vi "Write Voltage Data to Optimization.vi"(5 "Network Data Array":T1[](array[typedef]), 7 "Bus by ID":T2[](array[typedef]), 8 "error in":errorcluster, 11 "Generic Optimization in":refnum<class "Generic Optimization.lvclass">) -> (0 "error out":errorcluster, 3 "Generic Optimization out":refnum<class "Generic Optimization.lvclass">)   [LabVIEW 2018, in "Generic Optimization Actor.lvlib" / "Generic Optimization.lvclass"]
uses:
  Generic Optimization.lvclass
  C:/Users/Administrator/Desktop/LabVIEW EMS/EMS Generic Actor/EMS Generic/EMS Generic.lvclass
  Optimization Controls/Bus by ID.ctl
  <vilib>/ORNL/CSEISMIC DDS/CSEISMIC DDS Base/Data Types/Controls/DeviceID.ctl
  Optimization Controls/Electrical Network Optimization Data.ctl
  EMS Generic Actor/EMS Generic/EMS Generic.lvclass/EMS Generic.ctl
  Optimization Controls/Bus Voltage.ctl
  <vilib>/ORNL/CSEISMIC DDS/CSEISMIC DDS Base/Data Types/SmartRelay_Measurement.ctl
  <vilib>/ORNL/CSEISMIC DDS/CSEISMIC DDS Base/Data Types/DER_Measurement.ctl
  <vilib>/ORNL/CSEISMIC DDS/CSEISMIC DDS Base/Data Types/Meter_Measurement.ctl
  Global Variables/Global Variables.vi
  <vilib>/ORNL/CSEISMIC DDS/CSEISMIC DDS Base/CSEISMIC DDS.lvclass
  EMS Generic Actor/EMS Generic/EMS Generic.lvclass
  <vilib>/Analysis/NI_AALBase.lvlib
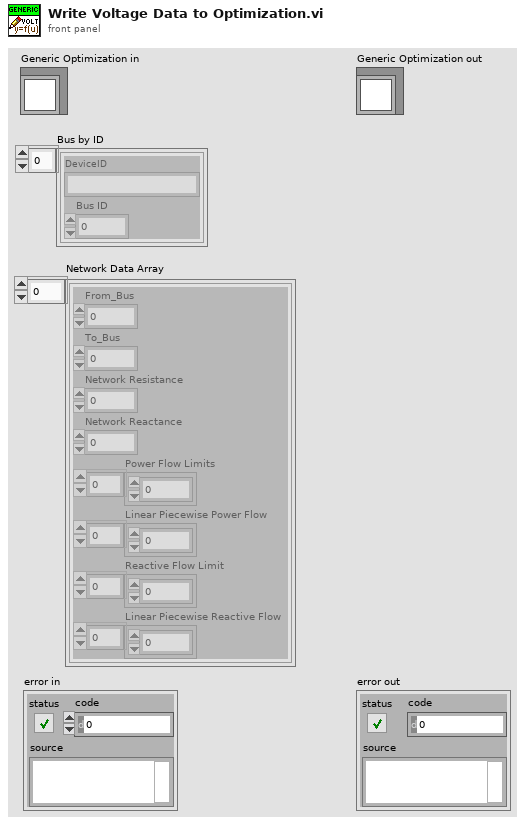
[diagram p1: front panel]
types:
  T1 = typedef "Generic Optimization Actor.lvlib/Generic Optimization.lvclass/Electrical Network Optimization Data.ctl" = cluster{"From_Bus":dbl, "To_Bus":dbl, "Network Resistance":dbl, "Network Reactance":dbl, "Power Flow Limits":dbl[], "Linear Piecewise Power Flow":dbl[], "Reactive Flow Limit":dbl[], "Linear Piecewise Reactive Flow":dbl[]}
  T2 = typedef "Generic Optimization Actor.lvlib/Generic Optimization.lvclass/Bus by ID.ctl" = cluster{"DeviceID":T3, "Bus ID":dbl}
  T3 = typedef "CSEISMIC DDS.lvlib/CSEISMIC DDS.lvclass/DeviceID.ctl" = string
  T4 = typedef "Generic Optimization Actor.lvlib/Generic Optimization.lvclass/Bus Voltage.ctl" = cluster{"Bus":dbl, "Voltage":dbl}
  T5 = typedef "CSEISMIC DDS.lvlib/CSEISMIC DDS.lvclass/Meter_Measurement.ctl" = cluster{"DeviceID":T3, "Voltage":dbl[], "Current":dbl[], "RealPower":dbl[], "ReactivePower":dbl[], "LineConfig":u8[], "Frequency":dbl}
  T6 = typedef "CSEISMIC DDS.lvlib/CSEISMIC DDS.lvclass/SmartRelay_Measurement.ctl" = cluster{"DeviceID":T3, "PrimaryVoltage":dbl[], "SecondaryVoltage":dbl[], "Current":dbl[], "RealPower":dbl[], "ReactivePower":dbl[], "LineConfig":u8[], "Frequency":dbl}
  T7 = typedef "CSEISMIC DDS.lvlib/CSEISMIC DDS.lvclass/DER_Measurement.ctl" = cluster{"DeviceID":T3, "Voltage":dbl[], "Current":dbl[], "RealPower":dbl[], "ReactivePower":dbl[], "LineConfig":u8[], "Frequency":dbl}
  T8 = typedef "EMS Generic Actor.lvlib/EMS Generic.lvclass/Data Type DVRs.ctl" = cluster{"IED_Status":refnum<data-value>, "IED_Status_0":refnum<data-value>, "DER_Measurement":refnum<data-value>, "DER_Info":refnum<data-value>, "DER_Status":refnum<data-value>, "ES_Measurement":refnum<data-value>, "ES_Info":refnum<data-value>, "PV_Info":refnum<data-value>, "SmartRelay_Info":refnum<data-value>, "SmartRelay_Measurement":refnum<data-value>, "Meter_Info":refnum<data-value>, "Meter_Measurement":refnum<data-value>, "HVAC_Status":refnum<data-value>, "HVAC_Measurement":refnum<data-value>, "PriceData_RealTime":refnum<data-value>, "PriceData_Demand":refnum<data-value>, "PriceData_Energy":refnum<data-value>, "ForecastData_Long":refnum<data-value>, "ForecastData_Short":refnum<data-value>, "DER_Control":refnum<data-value>, "DER_SetPointF":refnum<data-value>, "DER_SetPointP":refnum<data-value>, "DER_SetPointQ":refnum<data-value>, "DER_SetPointPF":refnum<data-value>, "DER_SetPointV":refnum<data-value>, "PV_setCurtailment":refnum<data-value>, "PV_setRampRate":refnum<data-value>, "Relay_Control":refnum<data-value>, "Load_Control":refnum<data-value>, "HVAC_Control":refnum<data-value>, "Generator_Info":refnum<data-value>, "ForecastData_Long_Backup":refnum<data-value>, "PriceData_RealTime_Backup":refnum<data-value>}
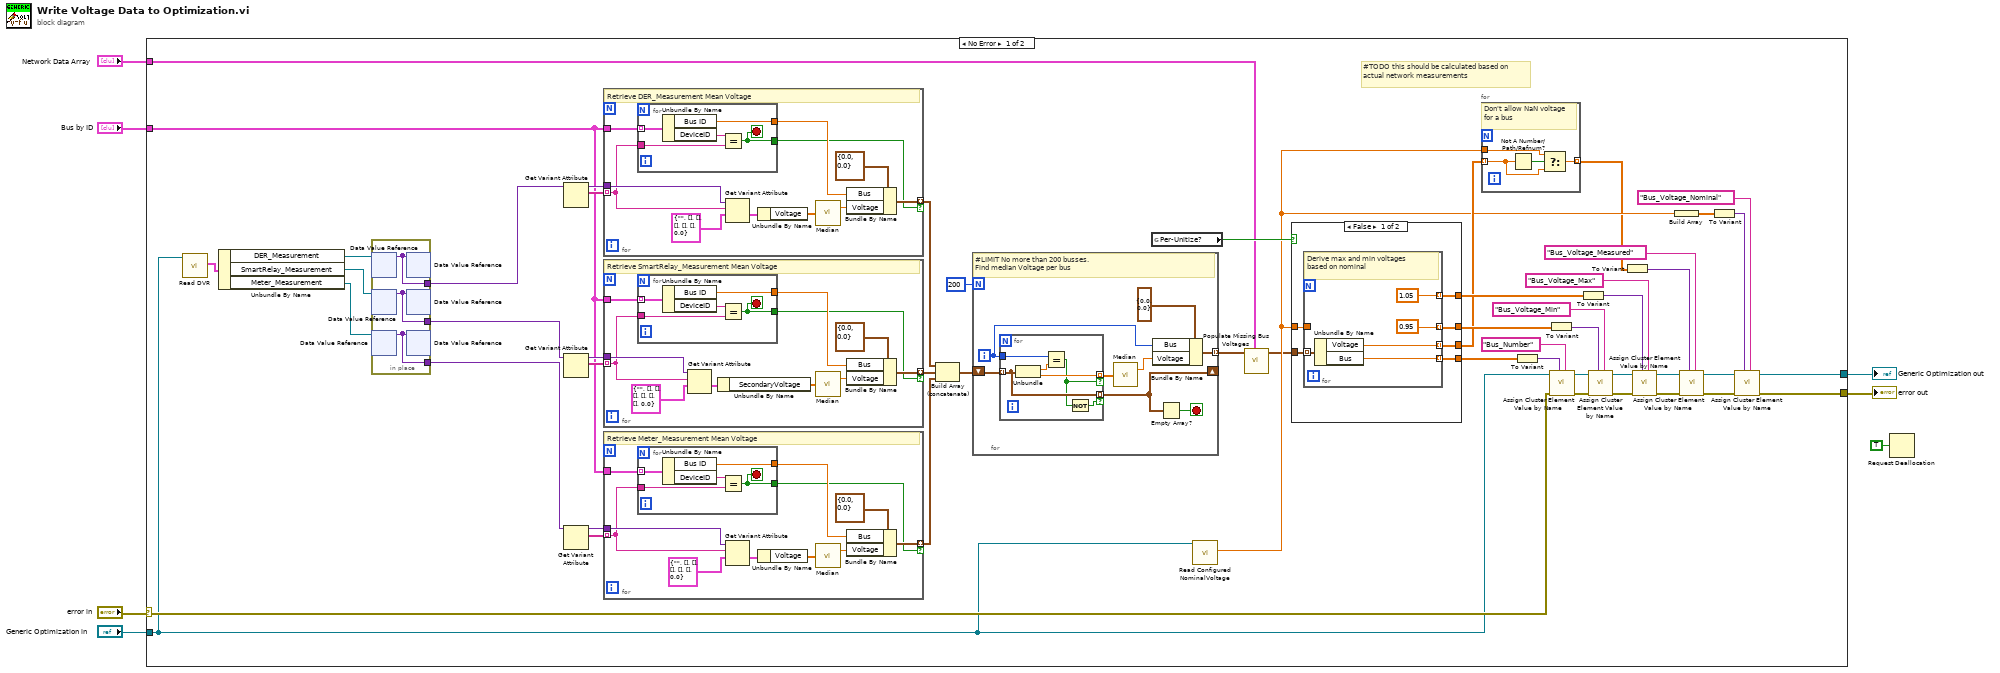
[diagram p0: block diagram]
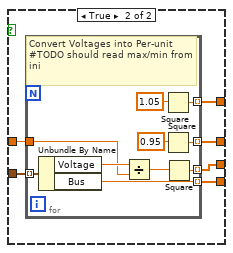
[diagram p2: hidden frame]
diagram:
  n1 = case shown="No Error" "error in" {
    selector: "error in" -> [w45 w157]
    tunnel: [w20 w157] -> w7
    tunnel: "Bus by ID" -> [w27 _]
    tunnel: "Generic Optimization in" -> [w9 w156]
    tunnel: [w8 w156] -> w3
    tunnel: "Network Data Array" -> [w10 _]
    frame No Error {
      # "#TODO this should be calculated based on actual network measurements"
      n2 = call "Read DVR.vi"("EMS Generic in"=w9) -> ("DVR"=w41:T8)  [unwired: 9 in, 1 out]
      n3 = Unbundle By Name(w41) -> ("DER_Measurement"=w40:refnum<data-value>, "SmartRelay_Measurement"=w39:refnum<data-value>, "Meter_Measurement"=w26:refnum<data-value>)
      n4 = in-place {
        in-place-border: [w155] -> w25
        in-place-border: [w154] -> w24
        in-place-border: [w153] -> w23
        n5 = in-place-dvr #1(w40) -> (w155:variant)  [unwired: 1 out]
        n6 = in-place-dvr #2(w39) -> (w154:variant)  [unwired: 1 out]
        n7 = in-place-dvr #3(w26) -> (w153:variant)  [unwired: 1 out]
        n8 = in-place-dvr #1(w155) -> ()  [unwired: 2 out]
        n9 = in-place-dvr #2(w154) -> ()  [unwired: 2 out]
        n10 = in-place-dvr #3(w153) -> ()  [unwired: 2 out]
      }
      n11 = Get Variant Attribute(Variant=w25) -> (duplicate Variant=w37:variant, names=w38:string[])  [unwired: 3 in, 2 out]
      n12 = Get Variant Attribute(Variant=w24) -> (duplicate Variant=w36:variant, names=w35:string[])  [unwired: 3 in, 2 out]
      n13 = Get Variant Attribute(Variant=w23) -> (duplicate Variant=w33:variant, names=w34:string[])  [unwired: 3 in, 2 out]
      n14 = for {
        tunnel: w38 -> [w145] mode=indexing
        tunnel: w37 -> [w147]
        tunnel: w27 -> [w146]
        tunnel: [w143] -> w32 mode=indexing if=w137
        # "Retrieve DER_Measurement Mean Voltage"
        n15 = for {
          tunnel: w146 -> [w152] mode=indexing
          tunnel: w145 -> [w151]
          tunnel: [w149] -> w139
          tunnel: [w148] -> w137
          stop <- w148 stop-if-true
          n16 = Unbundle By Name(w152) -> ("Bus ID"=w149:dbl, "DeviceID"=w150:T3)
          n17 = Equal?(x=w150, y=w151) -> (x = y?=w148:bool)
        }
        n18 = Get Variant Attribute(Variant=w147, name=w145, default value (empty Variant)=T7 {"DeviceID"="", "Voltage"=[], "Current"=[], "RealPower"=[], "ReactivePower"=[], "LineConfig"=[], "Frequency"=0.0} ("DER_Measurement")) -> (value=w144:T7)  [unwired: 1 in, 3 out]
        n19 = Unbundle By Name(w144) -> ("Voltage"=w141:dbl[])
        n20 = call <vilib>:"Median.vi"("X"=w141) -> ("median"=w140:dbl)  [unwired: 1 out]
        n21 = Bundle By Name(cluster=T4 {"Bus"=0.0, "Voltage"=0.0} ("Bus Voltage"), "Bus"=w139, "Voltage"=w140) -> (w143:T4)
      }
      n22 = for {
        tunnel: w35 -> [w129] mode=indexing
        tunnel: w36 -> [w131]
        tunnel: w27 -> [w130]
        tunnel: [w127] -> w31 mode=indexing if=w122
        # "Retrieve SmartRelay_Measurement Mean Voltage"
        n23 = for {
          tunnel: w130 -> [w136] mode=indexing
          tunnel: w129 -> [w135]
          tunnel: [w133] -> w124
          tunnel: [w132] -> w122
          stop <- w132 stop-if-true
          n24 = Unbundle By Name(w136) -> ("Bus ID"=w133:dbl, "DeviceID"=w134:T3)
          n25 = Equal?(x=w134, y=w135) -> (x = y?=w132:bool)
        }
        n26 = Get Variant Attribute(Variant=w131, name=w129, default value (empty Variant)=T6 {"DeviceID"="", "PrimaryVoltage"=[], "SecondaryVoltage"=[], "Current"=[], "RealPower"=[], "ReactivePower"=[], "LineConfig"=[], "Frequency"=0.0} ("SmartRelay_Measurement")) -> (value=w128:T6)  [unwired: 1 in, 3 out]
        n27 = Unbundle By Name(w128) -> ("SecondaryVoltage"=w126:dbl[])
        n28 = call <vilib>:"Median.vi"("X"=w126) -> ("median"=w125:dbl)  [unwired: 1 out]
        n29 = Bundle By Name(cluster=T4 {"Bus"=0.0, "Voltage"=0.0} ("Bus Voltage"), "Bus"=w124, "Voltage"=w125) -> (w127:T4)
      }
      n30 = for {
        tunnel: w34 -> [w113] mode=indexing
        tunnel: w33 -> [w115]
        tunnel: w27 -> [w114]
        tunnel: [w111] -> w30 mode=indexing if=w106
        # "Retrieve Meter_Measurement Mean Voltage"
        n31 = for {
          tunnel: w114 -> [w120] mode=indexing
          tunnel: w113 -> [w119]
          tunnel: [w117] -> w108
          tunnel: [w116] -> w106
          stop <- w116 stop-if-true
          n32 = Unbundle By Name(w120) -> ("Bus ID"=w117:dbl, "DeviceID"=w118:T3)
          n33 = Equal?(x=w118, y=w119) -> (x = y?=w116:bool)
        }
        n34 = Get Variant Attribute(Variant=w115, name=w113, default value (empty Variant)=T5 {"DeviceID"="", "Voltage"=[], "Current"=[], "RealPower"=[], "ReactivePower"=[], "LineConfig"=[], "Frequency"=0.0} ("Meter_Measurement")) -> (value=w112:T5)  [unwired: 1 in, 3 out]
        n35 = Unbundle By Name(w112) -> ("Voltage"=w110:dbl[])
        n36 = call <vilib>:"Median.vi"("X"=w110) -> ("median"=w109:dbl)  [unwired: 1 out]
        n37 = Bundle By Name(cluster=T4 {"Bus"=0.0, "Voltage"=0.0} ("Bus Voltage"), "Bus"=w108, "Voltage"=w109) -> (w111:T4)
      }
      n38 = Build Array (concatenate)(w32, w31, w30) -> (w29:T4[])
      n39 = for {
        N: 200 -> [_]
        shift-right: [w97] -> _
        shift-left: w29 -> [w98]
        tunnel: [w93] -> w12 mode=indexing
        i -> [w94]
        stop <- w96 stop-if-true
        # "#LIMIT No more than 200 busses.\nFind median Voltage per bus"
        n40 = for {
          tunnel: w98 -> [w101] mode=indexing
          tunnel: w94 -> [w104]
          tunnel: [w102] -> w92 mode=indexing if=w100
          tunnel: [w101] -> w97 mode=indexing if=w99
          n41 = Unbundle(w101) -> ("Bus"=w103:dbl, "Voltage"=w102:dbl)
          n42 = Equal?(x=w104, y=w103) -> (x = y?=w100:bool)
          n43 = Not(x=w100) -> (.not. x?=w99:bool)
        }
        n44 = call <vilib>:"Median.vi"("X"=w92) -> ("median"=w91:dbl)  [unwired: 1 out]
        n45 = Bundle By Name(cluster=T4 {"Bus"=0.0, "Voltage"=0.0} ("Bus Voltage"), "Bus"=w94, "Voltage"=w91) -> (w93:T4)
        n46 = Empty Array?(array=w97) -> (empty?=w96:bool)
      }
      n47 = global read "Global Variables.vi" "Per-Unitize?"() -> (w22:bool)
      n48 = call "Read Configured NominalVoltage.vi"("EMS Generic in"=w9) -> ("NominalVoltage"=w14:dbl)  [unwired: 8 in, 2 out]
      n49 = call "Populate Missing Bus Voltages.vi"("Network Data Array"=w10, "Bus Voltage Array in"=w12) -> ("Bus Voltage Array out"=w11:T4[])  [unwired: 8 in, 1 out]
      n50 = case shown="False" w22 {
        tunnel: [w69 w75] -> w44
        tunnel: [w68 w77] -> w43
        tunnel: [w67 w78] -> w42
        tunnel: [w66 w76] -> w15
        tunnel: w11 -> [w65 w79]
        tunnel: w14 -> [w64 w80]
        frame False {
          n51 = for {
            tunnel: w65 -> [w74] mode=indexing
            tunnel: [w72] -> w66 mode=indexing
            tunnel: w64 -> [_]
            tunnel: [1.05] -> w67 mode=indexing
            tunnel: [0.95] -> w68 mode=indexing
            tunnel: [w73] -> w69 mode=indexing
            # "Derive max and min voltages based on nominal"
            n52 = Unbundle By Name(w74) -> ("Voltage"=w72:dbl, "Bus"=w73:dbl)
          }
        }
        frame True {
          n53 = for {
            tunnel: w79 -> [w90] mode=indexing
            tunnel: [w89] -> w76 mode=indexing
            tunnel: w80 -> [w84]
            tunnel: [w88] -> w78 mode=indexing
            tunnel: [w87] -> w77 mode=indexing
            tunnel: [w86] -> w75 mode=indexing
            # "Convert Voltages into Per-unit\n#TODO should read max/min from ini"
            n54 = Unbundle By Name(w90) -> ("Voltage"=w85:dbl, "Bus"=w86:dbl)
            n55 = Divide(x=w85, y=w84) -> (x/y=w81:dbl)
            n56 = Square(x=1.05) -> (x^2=w88:dbl)
            n57 = Square(x=0.95) -> (x^2=w87:dbl)
            n58 = Square(x=w81) -> (x^2=w89:dbl)
          }
        }
      }
      n59 = for {
        tunnel: w15 -> [w62] mode=indexing
        tunnel: w14 -> [w61]
        tunnel: [w60] -> w13 mode=indexing
        # "Don't allow NaN voltage for a bus"
        n60 = Not A Number/Path/Refnum?(number/path/refnum=w62) -> (NaN/Path/Refnum?=w63:bool)
        n61 = Select(t=w61, s=w63, f=w62) -> (s? t:f=w60:dbl)
      }
      n62 = To Variant(anything=w44) -> (Variant=w46:variant)
      n63 = To Variant(anything=w43) -> (Variant=w48:variant)
      n64 = call "Assign Cluster Element Value by Name.vi"("Element Name"="Bus_Number" ("Keyword Name"), "Value"=w46, "error in"=w45, "Generic Optimization"=w9) -> ("error out"=w57:errorcluster, "Generic Optimization out"=w56:refnum<class "Generic Optimization.lvclass">)  [unwired: 6 in]
      n65 = To Variant(anything=w42) -> (Variant=w50:variant)
      n66 = call "Assign Cluster Element Value by Name.vi"("Element Name"="Bus_Voltage_Min" ("Keyword Name"), "Value"=w48, "error in"=w57, "Generic Optimization"=w56) -> ("error out"=w58:errorcluster, "Generic Optimization out"=w55:refnum<class "Generic Optimization.lvclass">)  [unwired: 6 in]
      n67 = To Variant(anything=w13) -> (Variant=w52:variant)
      n68 = call "Assign Cluster Element Value by Name.vi"("Element Name"="Bus_Voltage_Max" ("Keyword Name"), "Value"=w50, "error in"=w58, "Generic Optimization"=w55) -> ("error out"=w59:errorcluster, "Generic Optimization out"=w54:refnum<class "Generic Optimization.lvclass">)  [unwired: 6 in]
      n69 = Build Array(w14) -> (w16:dbl[])
      n70 = call "Assign Cluster Element Value by Name.vi"("Element Name"="Bus_Voltage_Measured" ("Keyword Name"), "Value"=w52, "error in"=w59, "Generic Optimization"=w54) -> ("error out"=w21:errorcluster, "Generic Optimization out"=w19:refnum<class "Generic Optimization.lvclass">)  [unwired: 6 in]
      n71 = To Variant(anything=w16) -> (Variant=w18:variant)
      n72 = call "Assign Cluster Element Value by Name.vi"("Element Name"="Bus_Voltage_Nominal" ("Keyword Name"), "Value"=w18, "error in"=w21, "Generic Optimization"=w19) -> ("error out"=w20:errorcluster, "Generic Optimization out"=w8:refnum<class "Generic Optimization.lvclass">)  [unwired: 6 in]
    }
    frame Error {
    }
  }
  "error out" <- w7
  "Generic Optimization out" <- w3
  n73 = Request Deallocation(TRUE ("flag")) -> ()
